vi "WPI_CANTalonSRX_ConfigEnabledLimits.vi"(0 "CAN Talon SRX Ref":T1={"DeviceStatus"={"status"=FALSE, "code"=0, "source"=""}, "Type"=enum."PWM", "PWM"={"PWM Channel"=enum."PWM 1", "DeadBand"={"Name"="", "maxPositivePwm"=0, "minPositivePwm"=0, "centerPwm"=0, "maxNegativePwm"=0, "minNegativePwm"=0, "angularRange"=0}}, "CAN"={"Device Number"=0, "SetOutput VI Ref"=variant(enum8{"Percent VBus", "Current", "Speed", "Position", "Voltage"} enum."Percent VBus"), "GetOutput VI Ref"=variant(refnum<k1> refnum), "Enable VI Ref"=variant(dbl 12.0), "Disable VI Ref"=variant(enum8{"Percent VBus", "Speed", "Position", "Slave", "Unchanged / Invalid", "Voltage Compensation", "Current", "Motion Profile"} enum."Percent VBus"), "Data"=variant}, "Invert"=FALSE}, 5 "Override Limit Switches":bool, 7 "Forward Limit Switch Enable":bool=TRUE, 9 "Reverse Limit Switch Enable":bool=TRUE, 11 "error in (no error)":errorcluster, 12 "Forward Soft Limit Enable":bool, 13 "Reverse Soft Limit Enable":bool) -> (4 "CAN Talon SRX Ref":T1={"DeviceStatus"={"status"=FALSE, "code"=0, "source"=""}, "Type"=enum."PWM", "PWM"={"PWM Channel"=enum."PWM 1", "DeadBand"={"Name"="", "maxPositivePwm"=0, "minPositivePwm"=0, "centerPwm"=0, "maxNegativePwm"=0, "minNegativePwm"=0, "angularRange"=0}}, "CAN"={"Device Number"=0, "SetOutput VI Ref"=variant(enum8{"Percent VBus", "Current", "Speed", "Position", "Voltage"} enum."Percent VBus"), "GetOutput VI Ref"=variant(refnum<k1> refnum), "Enable VI Ref"=variant(dbl 12.0), "Disable VI Ref"=variant(enum8{"Percent VBus", "Speed", "Position", "Slave", "Unchanged / Invalid", "Voltage Compensation", "Current", "Motion Profile"} enum."Percent VBus"), "Data"=variant}, "Invert"=FALSE}, 15 "error out":errorcluster)   [LabVIEW 2016]
doc: "Configure the enable state of the hardware limit switches and the soft limits."
uses:
  <vilib>/Rock Robotics/WPI/MotorControl/WPI_MotorControlDeviceRef.ctl
  <vilib>/Rock Robotics/WPI/MotorControl/WPI_MotorControlType.ctl
  <vilib>/Rock Robotics/SystemInterfaces/DIO/FPGA_DIOPWMChannel.ctl
  <vilib>/Rock Robotics/WPI/PWM/WPI_PWMDeadband.ctl
  <vilib>/Rock Robotics/WPI/ThirdParty/CanMotor/TalonSRX/WPI_CANTalonSRX_GlobalOps.ctl
  <vilib>/Rock Robotics/WPI/ThirdParty/CanMotor/TalonSRX/WPI_CANTalonSRX_Params.ctl
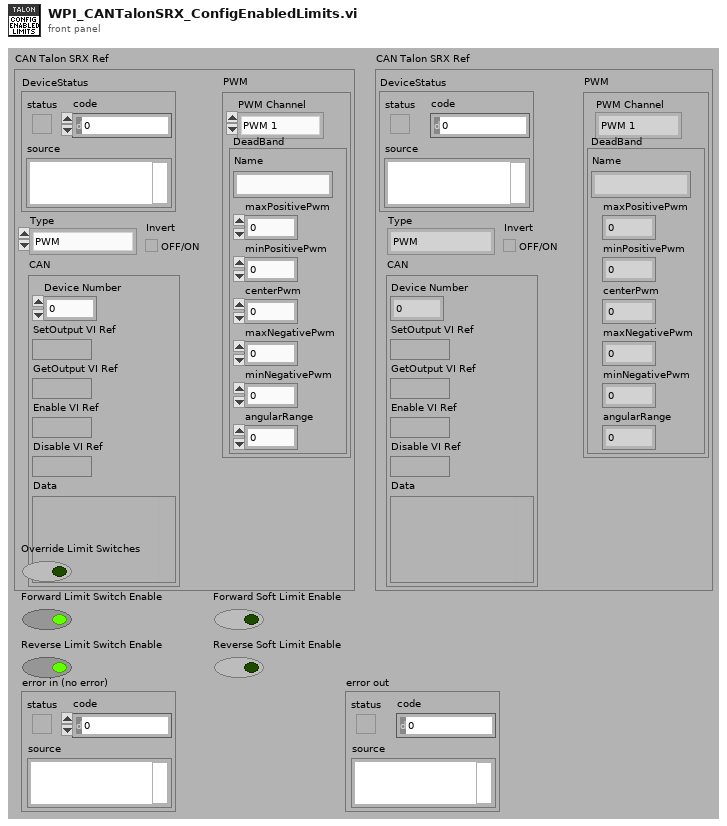
[diagram p1: front panel]
types:
  T1 = typedef "WPI_MotorControlDeviceRef.ctl" = cluster{"DeviceStatus":errorcluster, "Type":T2, "PWM":cluster{"PWM Channel":T3, "DeadBand":T4}, "CAN":cluster{"Device Number":u8, "SetOutput VI Ref":variant, "GetOutput VI Ref":variant, "Enable VI Ref":variant, "Disable VI Ref":variant, "Data":variant}, "Invert":bool}
  T2 = typedef "WPI_MotorControlType.ctl" = enum16{"PWM", "CAN"}
  T3 = typedef "FPGA_DIOPWMChannel.ctl" = enum8{"PWM 0", "PWM 1", "PWM 2", "PWM 3", "PWM 4", "PWM 5", "PWM 6", "PWM 7", "PWM 8", "PWM 9", "PWM MXP 0", "PWM MXP 1", "PWM MXP 2", "PWM MXP 3", "PWM MXP 4", "PWM MXP 5", "PWM MXP 6", "PWM MXP 7", "PWM MXP 8", "PWM MXP 9", "Invalid"}
  T4 = typedef "WPI_PWMDeadband.ctl" = cluster{"Name":string, "maxPositivePwm":i32, "minPositivePwm":i32, "centerPwm":i32, "maxNegativePwm":i32, "minNegativePwm":i32, "angularRange":u16}
  T5 = typedef "WPI_CANTalonSRX_GlobalOps.ctl" = enum16{"Read For Send", "Write After Receive General", "Write After Receive Feedback", "Write After Receive Encoder", "Write After Receive Ain", "Write Error", "Get All", "Set Output", "Set Mode", "Set Master ID", "Set Brake Mode", "Set Reverse Feedback Sensor", "Set Reverse Closed Loop Output", "Set Override Limits", "Set Forward Limit Enabled", "Set Reverse Limit Enabled", "Set Feedback Select", "Set Profile Select", "Set Throttle Ramp Rate", "Disable", "Set Enc Codes Per Rev", "Set Num Pot Turns", "Set Control Frame Rate", "Enable Legacy Control", "Write After Receive Pulse Width", "Set Enable Frame Rate", "Write After Receive Motion Profile", "Set Motion Profile Flow Control", "Set Motion Profile Control Frame Rate"}
  T6 = typedef "WPI_CANTalonSRX_Params.ctl" = u8
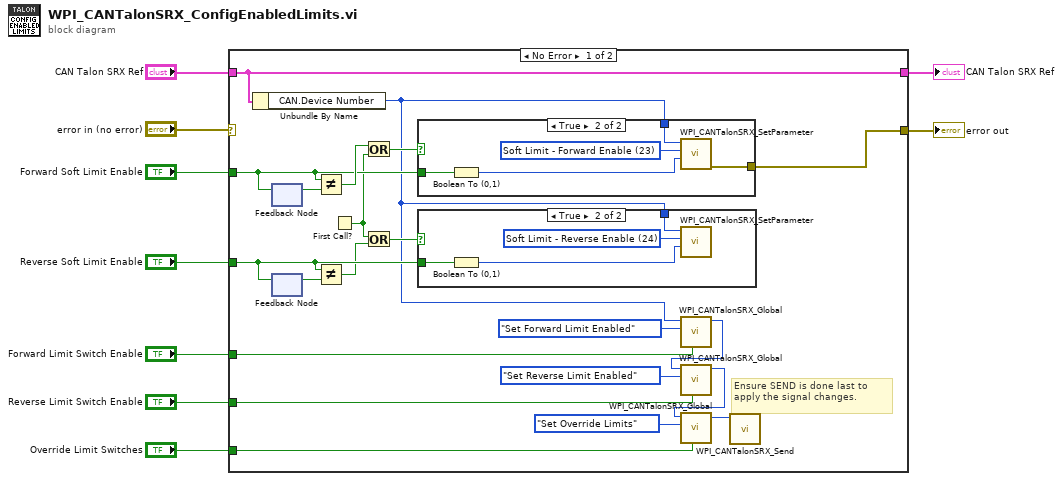
[diagram p0: block diagram]
diagram:
  n1 = case shown="No Error" "error in (no error)" {
    selector: "error in (no error)" -> [_ w41]
    tunnel: [w29 w41] -> w9
    tunnel: [w30 w40] -> w7
    tunnel: "CAN Talon SRX Ref" -> [w30 w40]
    tunnel: "Reverse Soft Limit Enable" -> [w21 _]
    tunnel: "Forward Soft Limit Enable" -> [w16 _]
    tunnel: "Reverse Limit Switch Enable" -> [w26 _]
    tunnel: "Forward Limit Switch Enable" -> [w25 _]
    tunnel: "Override Limit Switches" -> [w24 _]
    frame No Error {
      # "Ensure SEND is done last to apply the signal changes."
      n2 = Unbundle By Name(w30) -> ("CAN.Device Number"=w13:u8)
      n3 = feedback #1() -> (w17:bool)  [unwired: 1 in]
      n4 = feedback-in #1(w16) -> ()
      n5 = feedback-in #2(w21) -> ()
      n6 = feedback #2() -> (w22:bool)  [unwired: 1 in]
      n7 = Not Equal?(x=w16, y=w17) -> (x != y?=w18:bool)
      n8 = Not Equal?(x=w21, y=w22) -> (x != y?=w19:bool)
      n9 = First Call?() -> (First Call?: T/F=w15:bool)
      n10 = Or(x=w18, y=w15) -> (x .or. y?=w14:bool)
      n11 = Or(x=w15, y=w19) -> (x .or. y?=w20:bool)
      n12 = case shown="True" w14 {
        tunnel: w16 -> [_ w34]
        tunnel: [_ w32] -> w29
        tunnel: w13 -> [_ w31]
        frame False {
        }
        frame True {
          w35 = T6 23 items=["Slot 0 - P"=1, "Slot 0 - I"=2, "Slot 0 - D"=3, "Slot 0 - F"=4, "Slot 0 - I Zone"=5, "Slot 0 - Ramp Rate"=6, "Slot 1 - P"=11, "Slot 1 - I"=12, "Slot 1 - D"=13, "Slot 1 - F"=14, "Slot 1 - I Zone"=15, "Slot 1 - Ramp Rate"=16, "Soft Limit - Forward"=21, "Soft Limit - Reverse"=22, "Soft Limit - Forward Enable"=23, "Soft Limit - Reverse Enable"=24, "On Boot - Brake Mode"=31, "On Boot - Limit Normally Closed - Forward"=32, "On Boot - Limit Normally Closed - Reverse"=33, "On Boot - Limit Disabled - Forward"=34, "On Boot - Limit Disabled - Reverse"=35, "Fault - Over Temp"=41, "Fault - Under Voltage"=42, "Fault - Forward Limit"=43, "Fault - Reverse Limit"=44, "Fault - Hardware Failure"=45, "Fault - Forward Soft Limit"=46, "Fault - Reverse Soft Limit"=47, "Sticky Fault - Over Temp"=48, "Sticky Fault - Under Voltage"=49, "Sticky Fault - Forward Limit"=50, "Sticky Fault - Reverse Limit"=51, "Sticky Fault - Forward Soft Limit"=52, "Sticky Fault - Reverse Soft Limit"=53, "Applied Throttle"=61, "Closed-Loop Error"=62, "Select Feedback Device"=63, "Reverse Closed-Loop Output"=64, "Mode Select"=65, "Profile Slot Select"=66, "Ramp Throttle"=67, "Reverse Feedback Sensor"=68, "Limit Switch Enabled"=69, "Limit Switch Closed - Forward"=70, "Limit Switch Closed - Reverse"=71, "Sensor Position"=73, "Sensor Velocity"=74, "Current"=75, "Brake is Enabled"=76, "Encoder Position"=77, "Encoder Velocity"=78, "Encoder Index Rise Events"=79, "Encoder A Pin State"=80, "Encoder B Pin State"=81, "Encoder Index Pin State"=82, "Analog In with Overflow"=83, "Analog In Velocity"=84, "Temperature"=85, "Battery Voltage"=86, "Reset Count"=87, "Reset Flags"=88, "Firmware Version"=89, "Settings Changed"=90] ("Parameter")
          n13 = Boolean To (0,1)(Boolean=w34) -> (0, 1=w33:i16)
          n14 = call <vilib>:"WPI_CANTalonSRX_SetParameter.vi"("Value"=w33, "Parameter"=w35, "Device ID (0)"=w31) -> ("error out"=w32:errorcluster)  [unwired: 7 in, 1 out]
        }
      }
      n15 = case shown="True" w20 {
        tunnel: w21 -> [_ w38]
        tunnel: w13 -> [_ w36]
        frame False {
        }
        frame True {
          w39 = T6 24 items=["Slot 0 - P"=1, "Slot 0 - I"=2, "Slot 0 - D"=3, "Slot 0 - F"=4, "Slot 0 - I Zone"=5, "Slot 0 - Ramp Rate"=6, "Slot 1 - P"=11, "Slot 1 - I"=12, "Slot 1 - D"=13, "Slot 1 - F"=14, "Slot 1 - I Zone"=15, "Slot 1 - Ramp Rate"=16, "Soft Limit - Forward"=21, "Soft Limit - Reverse"=22, "Soft Limit - Forward Enable"=23, "Soft Limit - Reverse Enable"=24, "On Boot - Brake Mode"=31, "On Boot - Limit Normally Closed - Forward"=32, "On Boot - Limit Normally Closed - Reverse"=33, "On Boot - Limit Disabled - Forward"=34, "On Boot - Limit Disabled - Reverse"=35, "Fault - Over Temp"=41, "Fault - Under Voltage"=42, "Fault - Forward Limit"=43, "Fault - Reverse Limit"=44, "Fault - Hardware Failure"=45, "Fault - Forward Soft Limit"=46, "Fault - Reverse Soft Limit"=47, "Sticky Fault - Over Temp"=48, "Sticky Fault - Under Voltage"=49, "Sticky Fault - Forward Limit"=50, "Sticky Fault - Reverse Limit"=51, "Sticky Fault - Forward Soft Limit"=52, "Sticky Fault - Reverse Soft Limit"=53, "Applied Throttle"=61, "Closed-Loop Error"=62, "Select Feedback Device"=63, "Reverse Closed-Loop Output"=64, "Mode Select"=65, "Profile Slot Select"=66, "Ramp Throttle"=67, "Reverse Feedback Sensor"=68, "Limit Switch Enabled"=69, "Limit Switch Closed - Forward"=70, "Limit Switch Closed - Reverse"=71, "Sensor Position"=73, "Sensor Velocity"=74, "Current"=75, "Brake is Enabled"=76, "Encoder Position"=77, "Encoder Velocity"=78, "Encoder Index Rise Events"=79, "Encoder A Pin State"=80, "Encoder B Pin State"=81, "Encoder Index Pin State"=82, "Analog In with Overflow"=83, "Analog In Velocity"=84, "Temperature"=85, "Battery Voltage"=86, "Reset Count"=87, "Reset Flags"=88, "Firmware Version"=89, "Settings Changed"=90] ("Parameter")
          n16 = Boolean To (0,1)(Boolean=w38) -> (0, 1=w37:i16)
          n17 = call <vilib>:"WPI_CANTalonSRX_SetParameter.vi"("Value"=w37, "Parameter"=w39, "Device ID (0)"=w36) -> ()  [unwired: 7 in, 2 out]
        }
      }
      n18 = call <vilib>:"WPI_CANTalonSRX_Global.vi"("Set Boolean"=w25, "Operation"=WPI_CANTalonSRX_GlobalOps."Set Forward Limit Enabled", "Device ID (0)"=w13) -> ("Device ID Out"=w11:u8)  [unwired: 6 in, 2 out]
      n19 = call <vilib>:"WPI_CANTalonSRX_Global.vi"("Set Boolean"=w26, "Operation"=WPI_CANTalonSRX_GlobalOps."Set Reverse Limit Enabled", "Device ID (0)"=w11) -> ("Device ID Out"=w10:u8)  [unwired: 6 in, 2 out]
      n20 = call <vilib>:"WPI_CANTalonSRX_Global.vi"("Set Boolean"=w24, "Operation"=WPI_CANTalonSRX_GlobalOps."Set Override Limits", "Device ID (0)"=w10) -> ("Device ID Out"=w12:u8)  [unwired: 6 in, 2 out]
      n21 = call <vilib>:"WPI_CANTalonSRX_Send.vi"("Device ID (0)"=w12) -> ()  [unwired: 10 in, 1 out]
    }
    frame Error {
    }
  }
  "CAN Talon SRX Ref" <- w7
  "error out" <- w9
